vi "Test_Draw_To_Picture_ARGB.vi"(8 "error in (no error)":errorcluster) -> (0 "error out":errorcluster, 3 "Test Case Out":refnum<class "Image.lvclass">)   [LabVIEW 2020, in "g_ar_toolkit.test.lvlib" / "Image.lvclass"]
uses:
  Image.lvclass
  Image.lvclass/Image.ctl
  g_ar_toolkit.image/Image Size (Fixed).ctl
  g_ar_toolkit.image/g_ar_toolkit.image.lvlib
  g_ar_toolkit.image/Image Point (Fixed).ctl
  4993e8ee-a06a-463a-9684-69129f64d5ce.vi
panel:
  in  "Test Case in":refnum<class "Image.lvclass">
  out "Actual":picture
  out "Expected":picture
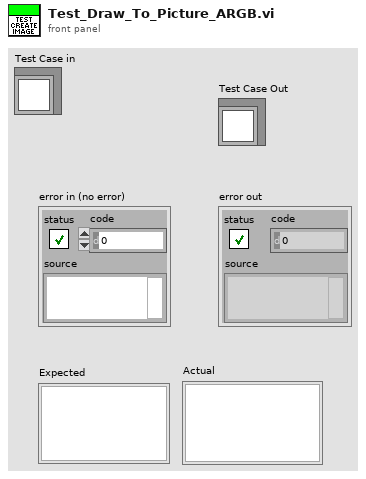
[diagram p1: front panel]
types:
  T1 = typedef "g_ar_toolkit.image.lvlib/Image Point (Fixed).ctl" = cluster{"x":i32, "y":i32}
  T2 = typedef "g_ar_toolkit.image.lvlib/Image Size (Fixed).ctl" = cluster{"Width":u16, "Height":u16}
  T3 = typedef "imagedata.ctl" = cluster{"image type":i32, "image depth":i32, "image":u8[], "mask":u8[], "colors":u32[], "Rectangle":cluster{"left":i16, "top":i16, "right":i16, "bottom":i16}}
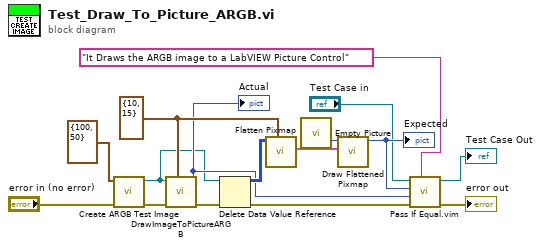
[diagram p0: block diagram]
diagram:
  w10 = T1 {"x"=10, "y"=15} ("Top-Left (0,0)")
  n1 = call "Create ARGB Test Image.vi"("error in (no error)"="error in (no error)", "Preallocated Image Size"=T2 {"Width"=100, "Height"=50} ("Preallocated Image Size (Default - 0,0)")) -> ("error out"=w2:errorcluster, "Data Value Reference out"=w1:refnum<data-value>)  [unwired: 7 in, 1 out]
  n2 = call "DrawImageToPictureARGB.vi"("Image Draw Offset (Default 0,0)"=w10, "error in (no error)"=w2, "ARGB Image Source"=w1) -> ("error out"=w11:errorcluster, "Picture"=w5:picture)  [unwired: 7 in]
  "Actual" <- w5
  n3 = Delete Data Value Reference(data value reference=w1, error in=w11) -> (data value=w7:u32[][], error out=w12:errorcluster)
  n4 = call <vilib>:"Flatten Pixmap.vi"("top left"=w10, "24-bit pixmap"=w7) -> ("image data"=w9:T3)  [unwired: 9 in]
  n5 = call "Empty Picture"() -> ("empty picture"=w8:picture)
  n6 = call <vilib>:"Draw Flattened Pixmap.vi"("image data"=w9, "picture"=w8) -> ("new picture"=w6:picture)  [unwired: 7 in]
  "Expected" <- w6
  n7 = call "Pass If Equal.vim"("Description"="It Draws the ARGB image to a LabVIEW Picture Control", "error in (no error)"=w12, "Actual"=w5, "Expected"=w6, "LUnit Test Case In"="Test Case in") -> ("error out"=→"error out":errorcluster, "LUnit Test Case Out"=→"Test Case Out":refnum<class "Image.lvclass">)  [unwired: 5 in]
